vi "array_raw_normalize.vi"(11 "array":u32[][](array[numeric])) -> (3 "Array":u8[][](array[numeric]))   [LabVIEW 2015]
uses:
  <vilib>/imath/engines/lvmath2/RunTimeEngine/BuiltInFunctions/int32/NIMS_int32(uint).vi
  <instcachedir>/0/NIMS_int32(uint)_312B4544F16B4D7EB378DAF313AFC32D.lvgen/NIMS_int32(uint)_312B4544F16B4D7EB378DAF313AFC32D_001.vi
  <vilib>/imath/engines/lvmath2/RunTimeEngine/BuiltInFunctions/abs/NIMS_abs(signed).vi
  <instcachedir>/0/NIMS_abs(signed)_C4FCB8E6058B49B797C7C8D53CA5F6EC.lvgen/NIMS_abs(signed)_C4FCB8E6058B49B797C7C8D53CA5F6EC_007.vi
  <vilib>/imath/engines/lvmath2/RunTimeEngine/NodeEndStatement/NIMS_NodeEndStatement_Output.vi
  <instcachedir>/0/NIMS_NodeEndStatement_Output_53EC0D466D134D7ABD903AC30B43404B.lvgen/NIMS_NodeEndStatement_Output_53EC0D466D134D7ABD903AC30B43404B_016.vi
  <vilib>/imath/engines/lvmath2/RunTimeEngine/ErrorHandling/NIMS_Finalize Error.vi
panel:
  out "array 2":u32[][](array[numeric]) format="%x"
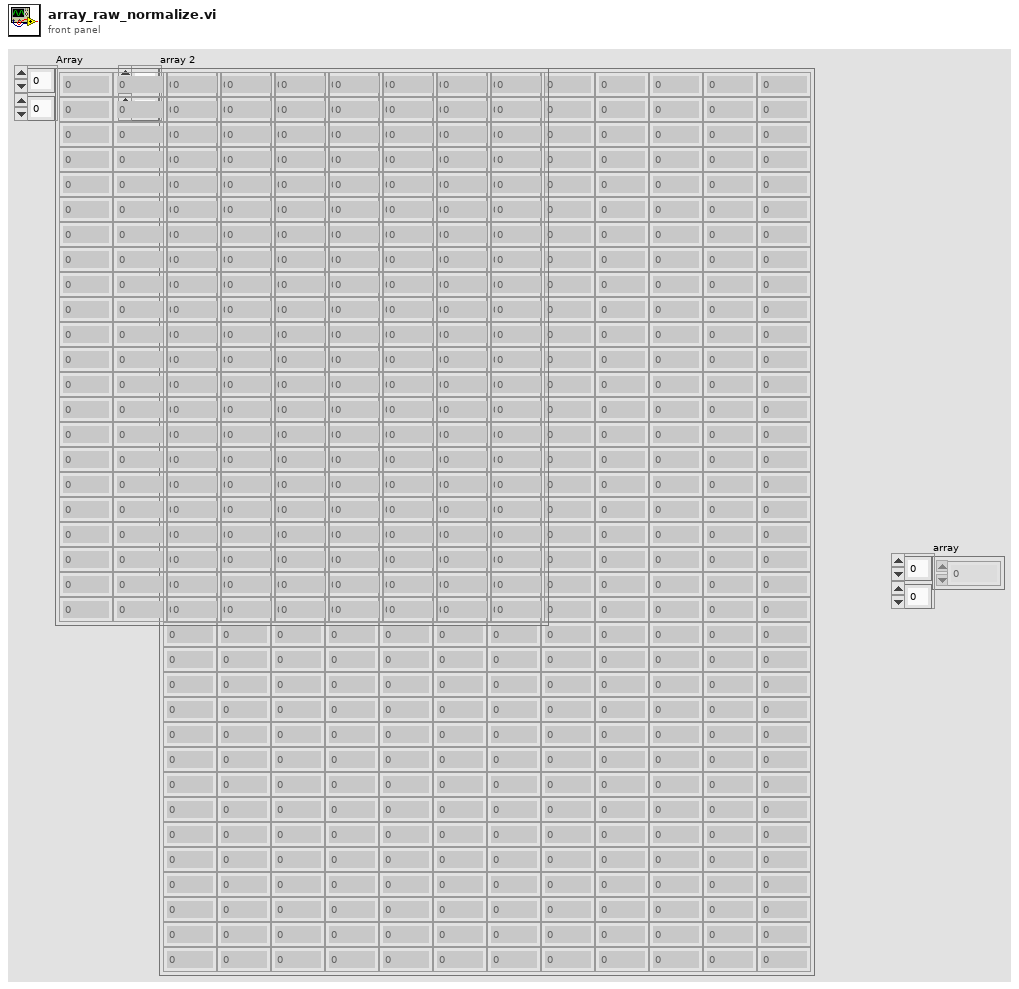
[diagram p1: front panel]
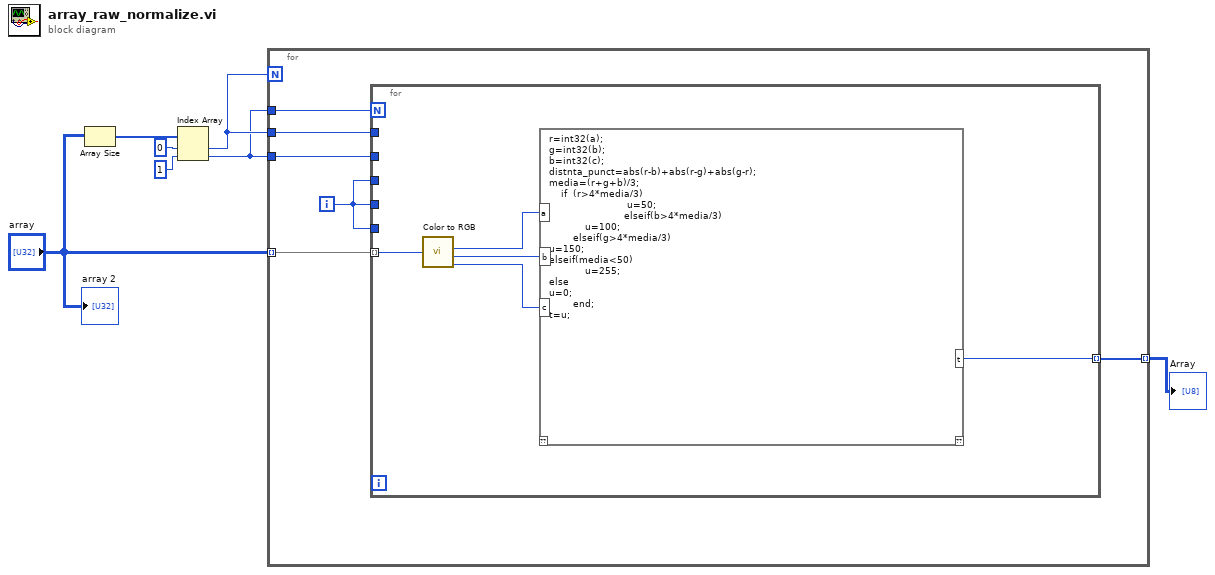
[diagram p0: block diagram]
diagram:
  n1 = Array Size(array="array") -> (size(s)=w7:i32[])
  n2 = Index Array(array=w7, index #1=0 ("index"), index #2=1 ("index")) -> (element #1=w4:i32, element #2=w3:i32)
  n3 = for {
    N: w4 -> [_]
    tunnel: w3 -> [w13]
    tunnel: "array" -> [w12] mode=indexing
    tunnel: w4 -> [w11]
    tunnel: w3 -> [w10]
    tunnel: [w8] -> w2 mode=indexing
    i -> [w9]
    n4 = for {
      N: w13 -> [_]
      tunnel: w12 -> [w17] mode=indexing
      tunnel: w9 -> [_]
      tunnel: w11 -> [_]
      tunnel: w10 -> [_]
      tunnel: w9 -> [_]
      tunnel: w9 -> [_]
      tunnel: [w14] -> w8 mode=indexing
      n5 = call <vilib>:"Color to RGB.vi"("Color"=w17) -> ("R"=w16:u8, "G"=w15:u8, "B"=w18:u8)  [unwired: 1 out]
      n6 = mathscript code="r=int32(a);\ng=int32(b);\nb=int32(c);\ndistnta_punct=abs(r-b)+abs(r-g)+abs(g-r);\nmedia=(r+g+b)/3;\n    if  (r>4*media/3)\n                          u=50;\n                         elseif(b>4*media/3)\n            u=100;\n        elseif(g>4*media/3)\nu=150;\nelseif(media<50)\n            u=255;\nelse\nu=0;\n        end;\nt=u;"("a"=w16, "b"=w15, "c"=w18) -> ("t"=w14:i32)  [unwired: 1 in, 1 out]
    }
  }
  "Array" <- w2
  "array 2" <- "array"
